vi "Configure External Modulation.vi"(5 "External Impedance (50: 50 Ohm)":i32(ring)=50 items=["50 Ohm"=50, "600 Ohm"=600, "1000000 Ohm"=1000000], 6 "External Coupling (0: AC)":i32(ring) items=["AC", "DC"], 7 "Modulation Source (1: External 1)":i32(ring)=1 items=["External 1"=1, "External 2"=2], 8 "error in (no error)":errorcluster, 9 "Modulation Path (1: 1)":i32(ring)=1 items=["1"=1, "2"=2], 10 "Modulation Type (0: Amplitude Modulation)":i32(ring) items=["Amplitude Modulation", "Frequency Modulation", "Phase Modulation"], 11 "VISA resource name":refnum<visa-resource-name>) -> (0 "error out":errorcluster, 3 "VISA resource name out":refnum<visa-resource-name>)   [LabVIEW 2012, in "Agilent PSG MXG Series.lvlib"]
doc: "Configures the external function generator source.\n\n<B>Notes:</B>\n(1) This VI is valid only inN5171B, N5172B, N5181B, N5182B that install <B>Option UNT</B> and <B>Option 303</B> (AM, FM, phase modulation, and LF output)."
uses:
  <instrlib>/Agilent PSG MXG Series/Agilent PSG MXG Series.lvlib
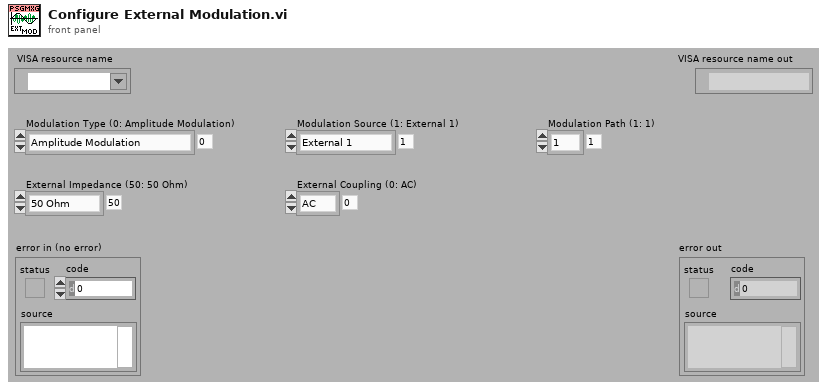
[diagram p1: front panel]
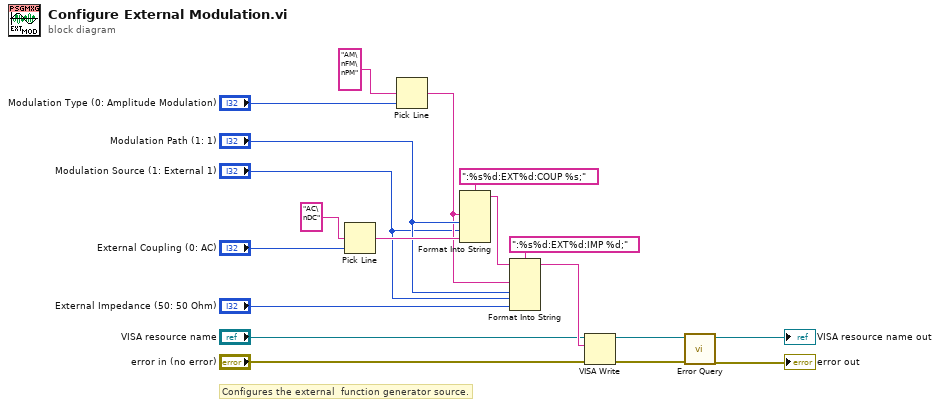
[diagram p0: block diagram]
diagram:
  # "Configures the external  function generator source."
  n1 = Pick Line(multi-line string="AC\nDC", line index="External Coupling (0: AC)") -> (output string=w6:string)  [unwired: 1 out]
  n2 = Pick Line(multi-line string="AM\nFM\nPM", line index="Modulation Type (0: Amplitude Modulation)") -> (output string=w2:string)  [unwired: 1 out]
  n3 = Format Into String(format string=":%s%d:EXT%d:COUP %s;", w2, "Modulation Path (1: 1)", "Modulation Source (1: External 1)", w6) -> (resulting string=w16:string)  [unwired: 2 in, 1 out]
  n4 = Format Into String(format string=":%s%d:EXT%d:IMP %d;", initial string=w16, w2, "Modulation Path (1: 1)", "Modulation Source (1: External 1)", "External Impedance (50: 50 Ohm)") -> (resulting string=w14:string)  [unwired: 1 in, 1 out]
  n5 = VISA Write(VISA resource name="VISA resource name", write buffer=w14, error in (no error)="error in (no error)") -> (VISA resource name out=w11:refnum<visa-resource-name>, error out=w10:errorcluster)  [unwired: 1 out]
  n6 = call <instrlib>:"Error Query.vi"("error in (no error)"=w10, "VISA resource name"=w11) -> ("error out"=→"error out":errorcluster, "VISA resource name out"=→"VISA resource name out":refnum<visa-resource-name>)  [unwired: 8 out]
